vi "GetState.vi"(8 "error in (no error)":errorcluster, 11 "reference in":refnum<class "Switch_Manager.lvclass">) -> (0 "error out":errorcluster, 1 "States":bool[](array[boolean]), 2 "Routes":string[](array[string]), 3 "reference in":refnum<class "Switch_Manager.lvclass">)   [LabVIEW 2022 SP3, in "Switch_Manager.lvlib" / "Switch_Manager.lvclass"]
uses:
  Switch_Manager.lvclass
  Components/SwitchBase.lvlibp/SwitchBase.lvclass
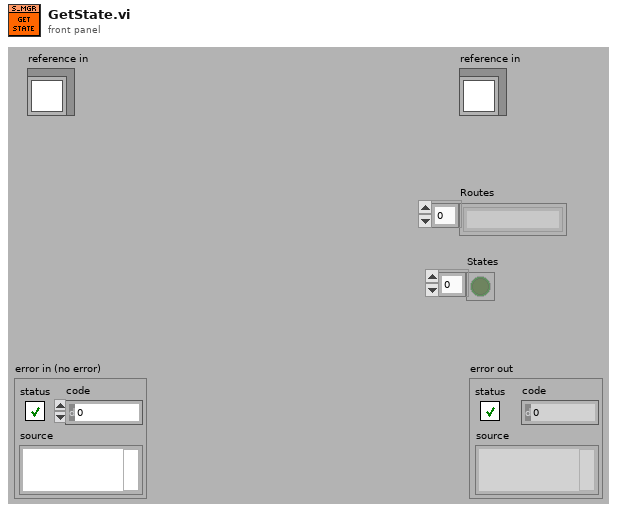
[diagram p1: front panel]
types:
  T1 = typedef "Switch_Manager.lvlib/Switch_Manager.lvclass/ObjectAttributes.ctl" = cluster{"Config":T2, "State":bool[], "Switches":refnum<class "SwitchBase.lvclass">[], "SwitchName":string[], "SwitchMap":T3[], "UpdateEvent":refnum<user-event>, "ParentEvent":refnum<user-event>, "Tree":bool[]}
  T2 = typedef "Switch_Manager.lvlib/Switch_Manager.lvclass/Config.ctl" = cluster{"default":string}
  T3 = typedef "Switch_Manager.lvlib/Switch_Manager.lvclass/SwitchMap.ctl" = cluster{"Name":string, "Description":string, "Group":string, "IsGroup":bool, "Switches":string[]}
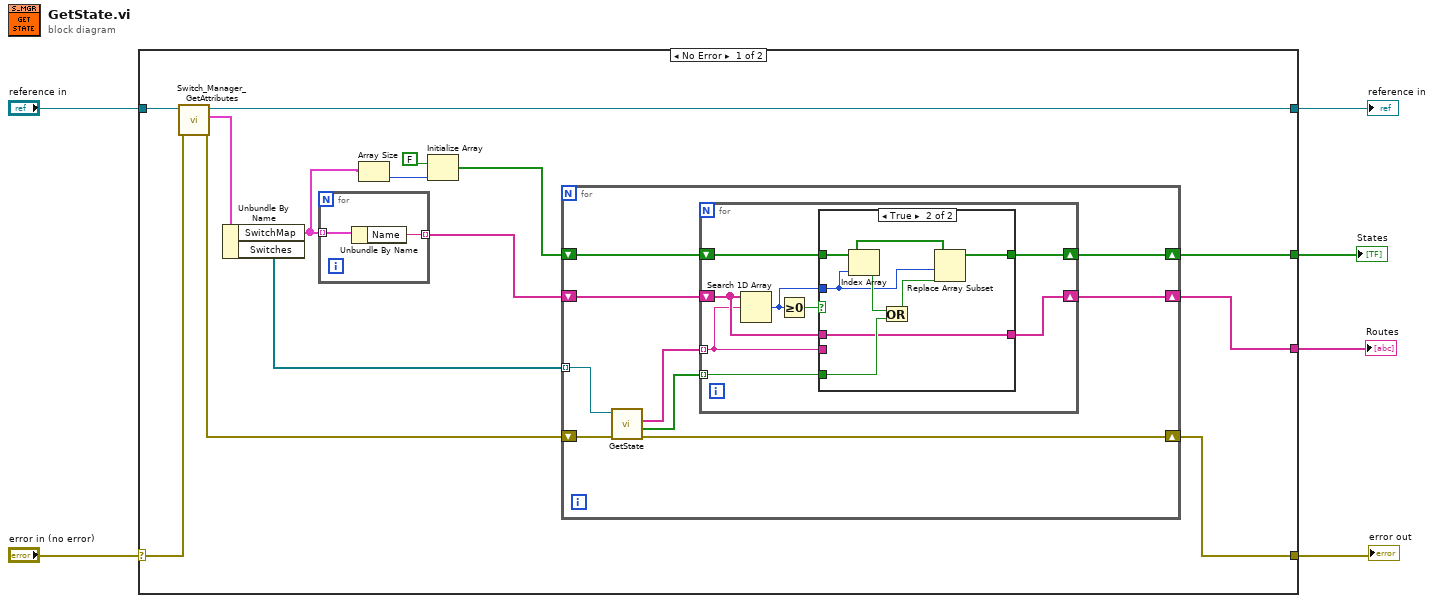
[diagram p0: block diagram]
diagram:
  n1 = case shown="No Error" "error in (no error)" {
    selector: "error in (no error)" -> [w20 w50]
    tunnel: [w14 w50] -> w5
    tunnel: [w18 w49] -> w3
    tunnel: "reference in" -> [w19 w49]
    tunnel: [w13 _] -> w2
    tunnel: [w12 _] -> w1
    frame No Error {
      n2 = call "Switch_Manager_GetAttributes.vi"("error in (no error)"=w20, "reference in"=w19) -> ("error out"=w15:errorcluster, "Data"=w17:T1, "reference out"=w18:refnum<class "Switch_Manager.lvclass">)  [unwired: 6 in, 1 out]
      n3 = Unbundle By Name(w17) -> ("SwitchMap"=w11:T3[], "Switches"=w16:refnum<class "SwitchBase.lvclass">[])
      n4 = for {
        tunnel: w11 -> [w22] mode=indexing
        tunnel: [w21] -> w8 mode=indexing
        n5 = Unbundle By Name(w22) -> ("Name"=w21:string)
      }
      n6 = Array Size(array=w11) -> (size(s)=w10:i32)
      n7 = Initialize Array(FALSE, w10) -> (w7:bool[])
      n8 = for {
        tunnel: w16 -> [w31] mode=indexing
        shift-right: [w29] -> w14
        shift-left: w15 -> [w30]
        shift-right: [w23] -> w13
        shift-left: w8 -> [w27]
        shift-right: [w24] -> w12
        shift-left: w7 -> [w25]
        n9 = call-dynamic "GetState.vi"("error in (no error)"=w30, "reference in"=w31) -> ("error out"=w29:errorcluster, "States"=w26:bool[], "Routes"=w28:string[])  [unwired: 6 in, 1 out]
        n10 = for {
          tunnel: w28 -> [w32] mode=indexing
          shift-right: [w33] -> w23
          shift-left: w27 -> [w34]
          tunnel: w26 -> [w39] mode=indexing
          shift-right: [w35] -> w24
          shift-left: w25 -> [w37]
          n11 = Search 1D Array(1D array=w34, element=w32) -> (index of element=w36:i32)  [unwired: 1 in]
          n12 = Greater Or Equal To 0?(x=w36) -> (x >= 0?=w38:bool)
          n13 = case shown="True" w38 {
            tunnel: w39 -> [_ w47]
            tunnel: w37 -> [w41 w46]
            tunnel: w36 -> [_ w44]
            tunnel: [w41 w43] -> w35
            tunnel: w34 -> [w40 w42]
            tunnel: [w40 w42] -> w33
            tunnel: w32 -> [_ _]
            frame False {
            }
            frame True {
              n14 = Index Array(array=w46, index=w44) -> (element=w48:bool)
              n15 = Or(x=w48, y=w47) -> (x .or. y?=w45:bool)
              n16 = Replace Array Subset(array=w46, new element=w45, index=w44) -> (w43:bool[])
            }
          }
        }
      }
    }
    frame Error {
    }
  }
  "error out" <- w5
  "reference in" <- w3
  "Routes" <- w2
  "States" <- w1
